vi "digital galvo ADC.vi"(10 "zero":dbl=32767.5 format="%#_13g", 11 "Analog waveform":dbl[](array[numeric])) -> (3 "Digital waveform":bool[](array[boolean]))   [LabVIEW 2015]
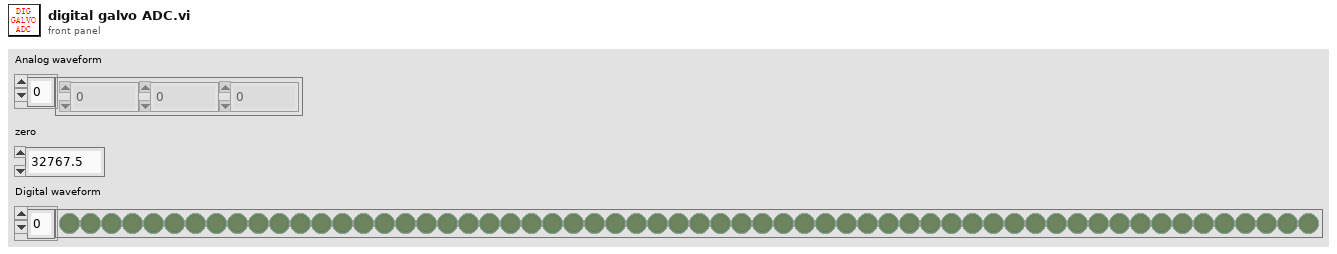
[diagram p1: front panel]
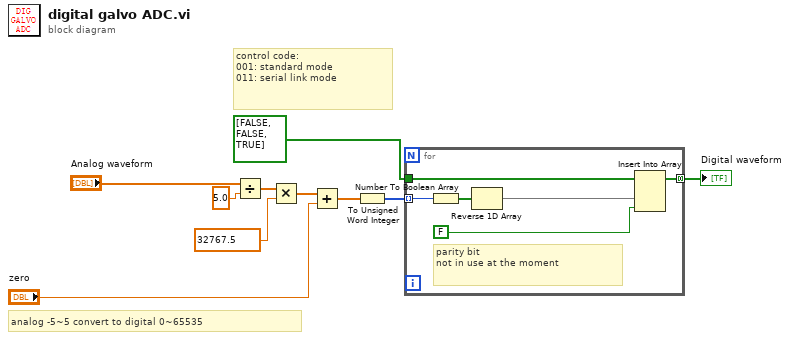
[diagram p0: block diagram]
diagram:
  # "analog -5~5 convert to digital 0~65535"
  # "control code:\n001: standard mode\n011: serial link mode"
  n1 = Divide(x="Analog waveform", y=5.0) -> (x/y=w9:dbl[])
  n2 = Multiply(x=w9, y=32767.5) -> (x*y=w8:dbl[])
  n3 = Add(x=w8, y="zero") -> (x+y=w6:dbl[])
  n4 = To Unsigned Word Integer(number=w6) -> (unsigned 16bit integer=w5:u16[])
  n5 = for {
    tunnel: w5 -> [w16] mode=indexing
    tunnel: bool[] [FALSE, FALSE, TRUE] ("Array") -> [w13]
    tunnel: [w11] -> w3 mode=concatenating
    # "parity bit\nnot in use at the moment"
    n6 = Number To Boolean Array(number=w16) -> (Boolean array=w15:bool[])
    n7 = Reverse 1D Array(array=w15) -> (reversed array=w14:bool[])
    n8 = Insert Into Array(array=w13, new element #1=w14, new element #2=FALSE ("new element/subarray")) -> (w11:bool[])  [unwired: 1 in]
  }
  "Digital waveform" <- w3
